vi "Exp_SetADCQuality.vi"(8 "error in (no error)":errorcluster, 10 "ADCQuality":T1 items=["LowNoise"=1, "HighCapacity"=2, "ElectronMultiplied"=3, "HighSpeed"=4], 11 "LightField Automation in":refnum<class "LightField Automation.lvclass">) -> (0 "error out":errorcluster, 3 "LightField Automation out":refnum<class "LightField Automation.lvclass">)   [LabVIEW 2015, in "LightField Automation.lvclass"]
uses:
  LightField Automation.lvclass
  TypeDefs/ADCQuality.ctl
  C:/Program Files/Princeton Instruments/LightField/PrincetonInstruments.LightFieldAddInSupportServices.dll
  Program Files/Princeton Instruments/LightField/PrincetonInstruments.LightFieldAddInSupportServices.dll
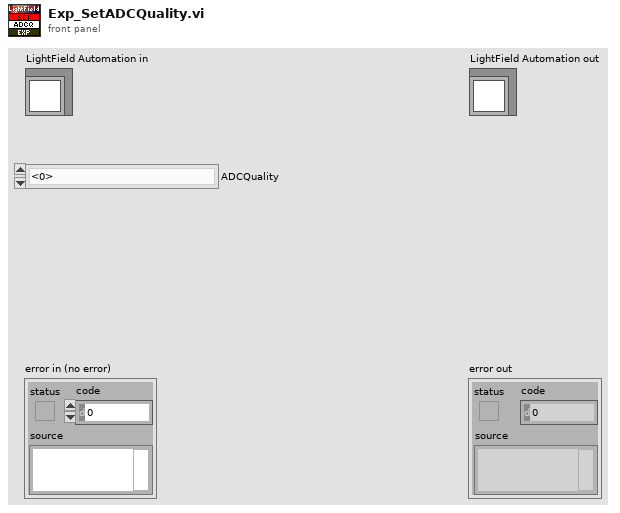
[diagram p1: front panel]
types:
  T1 = typedef "LightField Automation.lvclass/ADCQuality.ctl" = i32
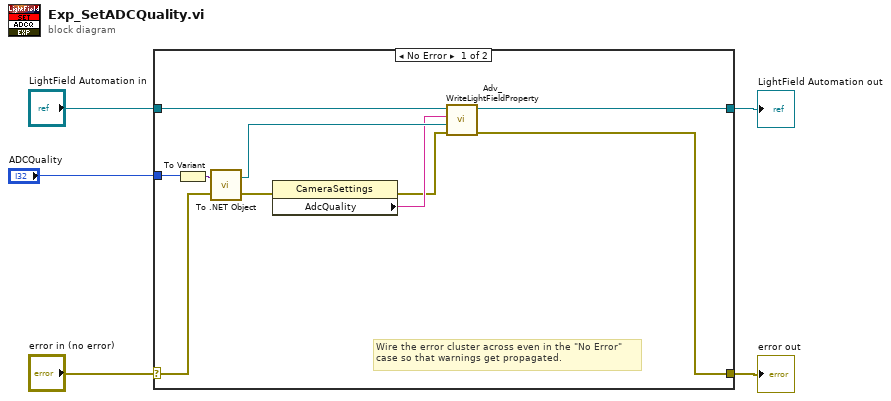
[diagram p0: block diagram]
diagram:
  n1 = case shown="No Error" "error in (no error)" {
    selector: "error in (no error)" -> [w11 w17]
    tunnel: [w6 w17] -> w4
    tunnel: [w14 w16] -> w2
    tunnel: "LightField Automation in" -> [w15 w16]
    tunnel: "ADCQuality" -> [w12 _]
    frame No Error {
      # "Wire the error cluster across even in the \"No Error\"\ncase so that warnings get propagated."
      n2 = To Variant(anything=w12) -> (Variant=w13:variant)
      n3 = call <vilib>:"To .NET Object.vi"("error in (no error)"=w11, "anything"=w13) -> ("error out"=w10:errorcluster, ".NET object"=w9:refnum<k24>)
      n4 = property class="CameraSettings"(error in=w10) -> (error out=w7:errorcluster, "AdcQuality"=w8:string)  [unwired: 1 in, 1 out]
      n5 = call "Adv_WriteLightFieldProperty.vi"("error in (no error)"=w7, "value"=w9, "setting"=w8, "LightField Automation in"=w15) -> ("error out"=w6:errorcluster, "LightField Automation out"=w14:refnum<class "LightField Automation.lvclass">)  [unwired: 6 in]
    }
    frame Error {
    }
  }
  "error out" <- w4
  "LightField Automation out" <- w2
